vi "Initialize Sessions - 1Sess.vi"(6 "initialize and close session behavior":T1, 8 "error in":errorcluster, 11 "session reservation in":refnum<class "Session Reservation.lvclass">) -> (0 "error out":errorcluster, 1 "channel list":string, 2 "session":string, 3 "session reservation out":refnum<class "Session Reservation.lvclass">)   [LabVIEW 2026, in "Session Management flexrio 148x.lvlib"]
uses:
  Session Management flexrio 148x.lvlib
  2ad95d60-3a16-4f23-aed6-967a0ffd0910.vi
  Session Factory/Session Factory.lvclass
  <vilib>/Plug-In SDKs/Clients/Session Management V1/Session Reservation/Session Reservation.lvclass
  <vilib>/Plug-In SDKs/Clients/Session Management V1/Session Reservation/Initialize and Close Session Behavior.ctl
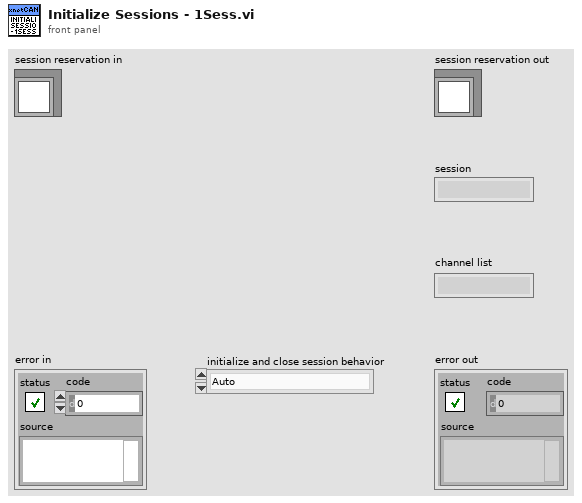
[diagram p1: front panel]
types:
  T1 = typedef "NI Session Management V1 Client.lvlib/Session Reservation.lvclass/Initialize and Close Session Behavior.ctl" = enum16{"Auto", "Initialize and Close", "Attach and Detach", "Initialize and Detach", "Attach and Close"}
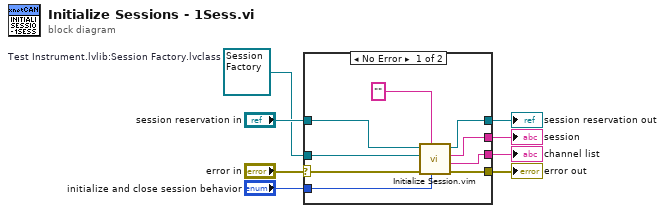
[diagram p0: block diagram]
diagram:
  w1 = refnum<class "Session Factory.lvclass"> refnum  # Test Instrument.lvlib:Session Factory.lvclass
  n1 = case shown="No Error" "error in" {
    selector: "error in" -> [w11 w19]
    tunnel: [w16 w19] -> w7
    tunnel: [w17 w18] -> w5
    tunnel: "session reservation in" -> [w13 w18]
    tunnel: [w15 _] -> w4
    tunnel: [w14 _] -> w3
    tunnel: "initialize and close session behavior" -> [w12 _]
    tunnel: w1 -> [w10 _]
    frame No Error {
      n2 = call "Initialize Session.vim"("initialize and close session behavior"=w12, "session type"="", "error in"=w11, "session factory"=w10, "session reservation in"=w13) -> ("error out"=w16:errorcluster, "channel list"=w15:string, "session"=w14:string, "session reservation out"=w17:refnum<class "Session Reservation.lvclass">)  [unwired: 3 in]
    }
    frame Error {
    }
  }
  "error out" <- w7
  "session reservation out" <- w5
  "channel list" <- w4
  "session" <- w3
